vi "kvCanSetBusParamsC200.vi"(0 "tseg1 - 2":u8 max=15 step=1, 1 "tseg2 - 1":u8 max=7 step=1, 2 "Ring":u8(ring) items=["1 Sample", "3 Samples"], 5 "error in (no error)":errorcluster, 6 "Prescaler - 1":u8 max=63 step=1, 7 "SJW - 1":u8 max=3 step=1, 8 "Channel Handle (input only)":i32) -> (3 "Channel Handle (ouput only)":i32, 4 "error out":errorcluster)   [LabVIEW 2022 SP3]
doc: "This function sets the bus timing parameters using the same convention as the 82c200 CAN controller (which is the same as many other CAN controllers, for example, the 82527.)\n\nNOTE: CANLIB32 will assume that the clock frequency is 16 MHz"
uses:
  canlib32.dll
panel:
  # "BTR0 Register"
  # "BTR1 Register"
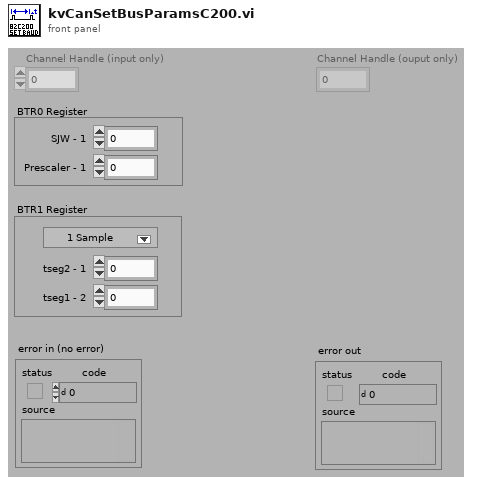
[diagram p1: front panel]
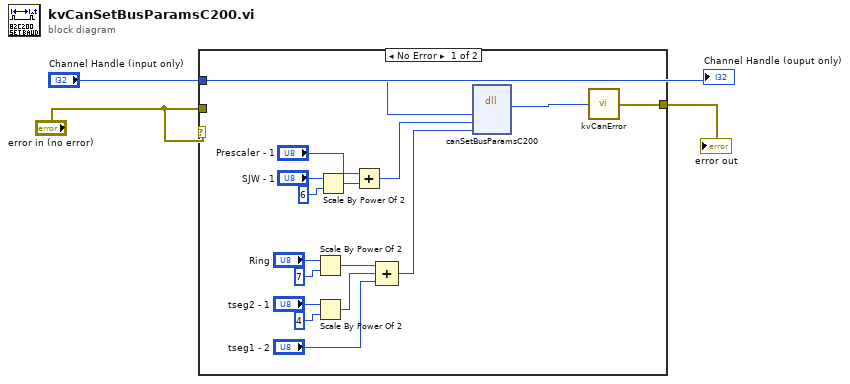
[diagram p0: block diagram]
diagram:
  n1 = case shown="No Error" "error in (no error)" {
    tunnel: [w19 w20] -> w3
    tunnel: "error in (no error)" -> [_ w20]
    tunnel: "Channel Handle (input only)" -> [w17 _]
    frame No Error {
      n2 = Scale By Power Of 2(n="Ring", x=7) -> (x*2^n=w7:i32)
      n3 = Scale By Power Of 2(n="tseg2 - 1", x=4) -> (x*2^n=w6:i32)
      n4 = Scale By Power Of 2(n="SJW - 1", x=6) -> (x*2^n=w14:i32)
      n5 = Add(x="Prescaler - 1", y=w14) -> (x+y=w12:i32)
      n6 = Compound Arithmetic op=ADD(w7, w6, "tseg1 - 2") -> (w4:i32)
      n7 = dll-call lib="canlib32.dll" fn="canSetBusParamsC200" label="Call canSetBusParamsC200"("channelHandle"=w17, "btr0"=w12, "btr1"=w4) -> (w18:i32)  [unwired: 6 in, 2 out]
      n8 = call "kvCanError.vi"("error code"=w18) -> ("error out"=w19:errorcluster)
    }
    frame Error {
    }
  }
  "error out" <- w3
  "Channel Handle (ouput only)" <- "Channel Handle (input only)"
